vi "VIPT to rename.vi"(11 "Package Source Folder":path) -> (0 "error out":errorcluster)   [LabVIEW 2019]
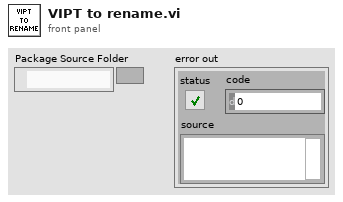
[diagram p1: front panel]
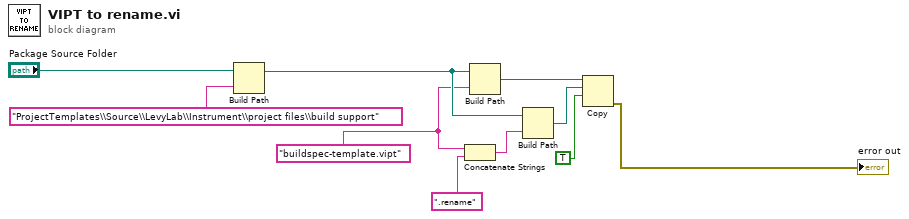
[diagram p0: block diagram]
diagram:
  w3 = "buildspec-template.vipt" ("name or relative path")
  n1 = Build Path(base path="Package Source Folder", name or relative path="ProjectTemplates\\Source\\LevyLab\\Instrument\\project files\\build support") -> (appended path=w7:path)
  n2 = Concatenate Strings(w3, ".rename" ("name or relative path")) -> (w2:string)
  n3 = Build Path(base path=w7, name or relative path=w3) -> (appended path=w8:path)
  n4 = Build Path(base path=w7, name or relative path=w2) -> (appended path=w6:path)
  n5 = Copy(9:TRUE ("overwrite (F)"), 10:w6, 11:w8) -> (0:→"error out":errorcluster)  [unwired: 2 in, 2 out]
